vi "S2C_FORNAX_Poly_BoardIdCommand.vi"(8 "Error In":errorcluster, 10 "BoardIdCommand":T4={"Partition"="Default", "Message"="BoardIdCommand", "M_BoardId"=0, "M_BoardIdDataSet"=0, "M_Command"=0, "M_Value"=""} {"M_Command" items=["BOARD_ID_COMMAND_NONE", "BOARD_ID_COMMAND_WRITE", "BOARD_ID_COMMAND_READ"]; "M_BoardIdDataSet" items=["BOARD_ID_DATASET_BOARD_INFO"=0, "BOARD_ID_DATASET_SCHEMA_INFO"=1, "BOARD_ID_DATASET_CHASSIS_INSTALLATION"=2, "BOARD_ID_DATASET_CONFIGURATION"=3, "BOARD_ID_DATASET_CALIBRATION_CURR"=4, "BOARD_ID_DATASET_RESERVED_1"=5, "BOARD_ID_DATASET_RESERVED_2"=6, "BOARD_ID_DATASET_RESERVED_3"=7, "BOARD_ID_DATASET_CALIBRATION_HIST_TOC"=8, "BOARD_ID_DATASET_CALIBRATION_HIST"=9, "BOARD_ID_DATASET_INIT_MAX"=10, "BOARD_ID_DATASET_MAX"=50]; "M_BoardId" items=["BOARD_ID_NONE", "BOARD_ID_CONTROLLER", "BOARD_ID_STEERING_RELAY", "BOARD_ID_RF", "BOARD_ID_POWER_SUPPLY", "BOARD_ID_FRONT_PANEL", "BOARD_ID_MAX"]}, 11 "Settings":T5={"Driver"="Fornax", "Command"="BoardIdCommand", "Return"="ErrorStatus", "Parameters"="", "Timeout"=10.0}) -> (0 "Error Out":errorcluster, 3 "Response":string)   [LabVIEW 2015]
uses:
  Typedefs/BoardId.ctl
  Typedefs/BoardIdDataSet.ctl
  Typedefs/BoardIdCommand.ctl
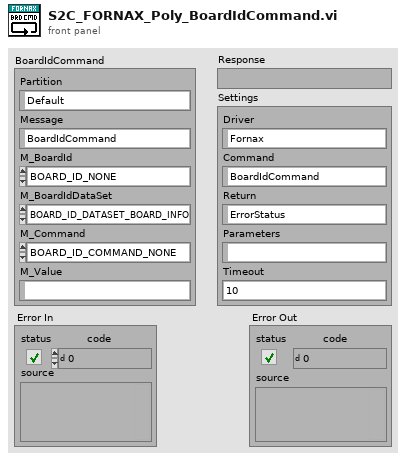
[diagram p1: front panel]
types:
  T1 = typedef "BoardId.ctl" = i16
  T2 = typedef "BoardIdDataSet.ctl" = i16
  T3 = typedef "BoardIdCommand.ctl" = i16
  T4 = cluster{"Partition":string, "Message":string, "M_BoardId":T1, "M_BoardIdDataSet":T2, "M_Command":T3, "M_Value":string}
  T5 = cluster{"Driver":string, "Command":string, "Return":string, "Parameters":string, "Timeout":dbl}
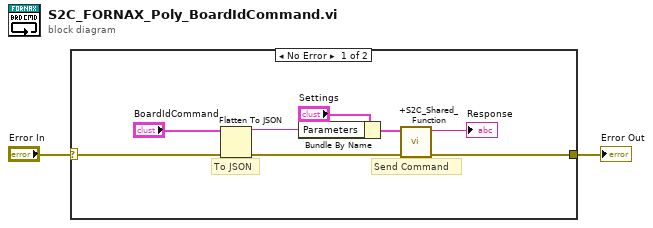
[diagram p0: block diagram]
diagram:
  n1 = case shown="No Error" "Error In" {
    selector: "Error In" -> [w6 w11]
    tunnel: [w5 w11] -> w1
    frame No Error {
      # "To JSON"
      # "Send Command"
      n2 = Flatten To JSON(anything="BoardIdCommand", error in (no error)=w6) -> (JSON string=w7:string, 11:w9:errorcluster)  [unwired: 1 in]
      n3 = Bundle By Name(cluster="Settings", "Parameters"=w7) -> (w10:T5)
      n4 = call "+S2C_Shared_Function.vi"("Error In"=w9, "Settings"=w10) -> ("Error Out"=w5:errorcluster, "Response"=→"Response":string)  [unwired: 8 in]
    }
    frame Error {
    }
  }
  "Error Out" <- w1
